vi "Lockin_Metrics.vi"() -> ()   [LabVIEW 2019]
uses:
  src/Instrument.DAQ/Typedefs/DAQ.Sampling.Sampling--Cluster.ctl
  src/Instrument.Lockin/Instrument.Lockin.lvclass
  src/Instrument.Lockin/Typedefs/Results Type--Enum.ctl
  src/Instrument.DAQ/Instrument.DAQ.lvclass
panel:
  in  "Fs":dbl[](array[numeric])=[204800.0, 180000.0, 160000.0, 140000.0, 120000.0, 102400.0, 90000.0, 80000.0, 70000.0, 60000.0, 51200.0, 40000.0, 30000.0, 25600.0, 20000.0, 15000.0, 12800.0]
  out "N":i32=97280
  out "XY Graph 4":cluster{dbl[], dbl[]}[](graph)
  out "XY Graph 3":cluster{dbl[], i32[]}[](graph)
  in  "N start":dbl=102400.0
  in  "N end":dbl=20480.0
  in  "N step":dbl=5120.0
  out "XY Graph 2":cluster{i32[], dbl[]}[](graph)
  in  "stop":bool
  out "Frequency (Hz)":dbl=100.0
  out "XY Graph":cluster{dbl[], dbl[]}[](graph)
  in  "f step":dbl=0.1
  in  "f end":dbl=3.5
  in  "f start":dbl=3.3
  # "Sweep frequency:"
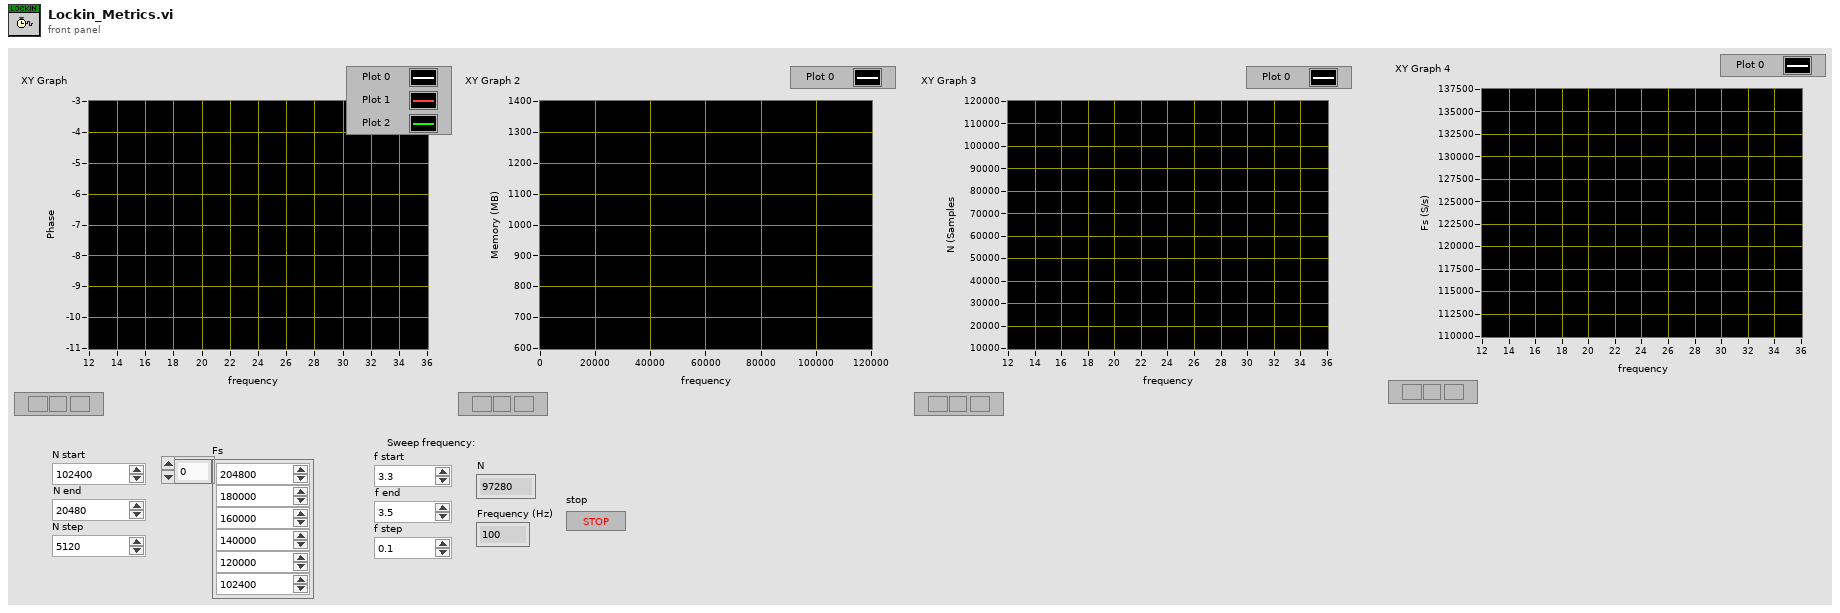
[diagram p1: front panel]
types:
  T1 = typedef "Instrument.Lockin.lvlib/Instrument.DAQ.lvclass/DAQ.Sampling.Sampling--Cluster.ctl" = cluster{"Fs":dbl, "#s":i32}
  T2 = typedef "Instrument.Lockin.lvlib/Instrument.Lockin.lvclass/Results Type--Enum.ctl" = enum16{"X", "Y", "R", "Theta", "Mean"}
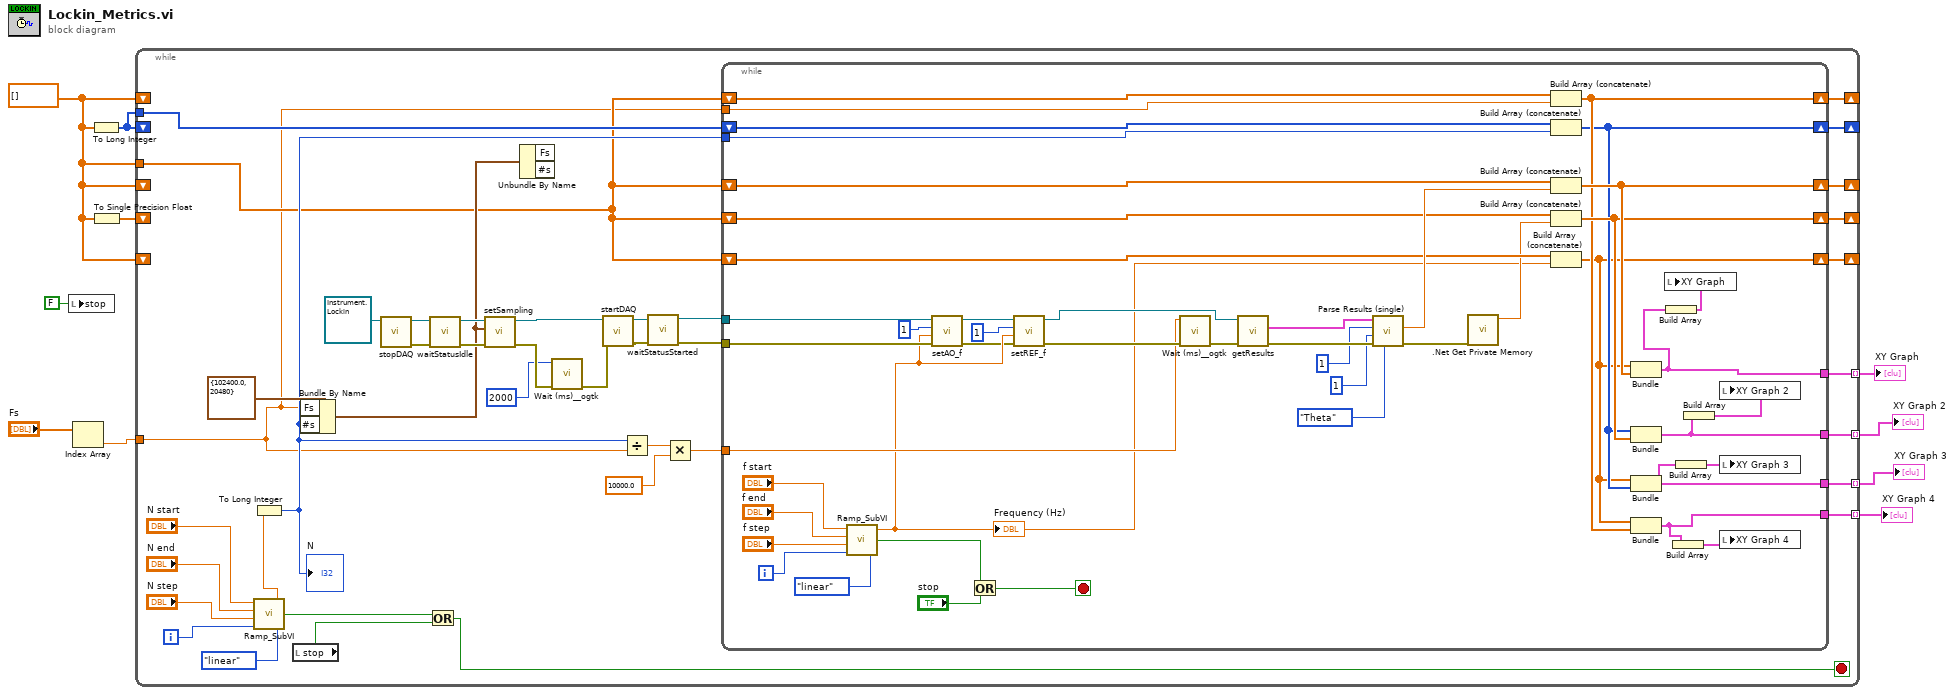
[diagram p0: block diagram]
diagram:
  w7 = dbl[] []
  n1 = local write "stop"(FALSE ("stop")) -> ()
  n2 = Index Array(array="Fs") -> (element=w5:dbl)  [unwired: 1 in]
  n3 = To Long Integer(number=w7) -> (32bit integer=w1:i32[])
  n4 = To Single Precision Float(number=w7) -> (single precision float=w9:sgl[])
  n5 = while {
    shift-right: [w42] -> _
    shift-left: w7 -> [_]
    shift-right: [w39] -> _
    shift-left: w1 -> [_]
    shift-right: [w38] -> _
    shift-left: w7 -> [_]
    shift-right: [w40] -> _
    shift-left: w7 -> [_]
    shift-right: [w41] -> _
    shift-left: w9 -> [_]
    tunnel: [w37] -> w8 mode=indexing
    tunnel: w7 -> [w15]
    tunnel: w5 -> [w14]
    tunnel: [w19] -> w2 mode=indexing
    tunnel: [w18] -> w3 mode=indexing
    tunnel: [w17] -> w4 mode=indexing
    tunnel: w1 -> [w16]
    i -> [w46]
    stop <- w36 stop-if-true
    n6 = call <userlib>:"Ramp_SubVI.vi"("Enum"=enum16{"linear", "power"}."linear", "index"=w46, "step"="N step", "end"="N end", "start"="N start") -> ("Stop?"=w45:bool, "Numeric"=w32:dbl)
    n7 = To Long Integer(number=w32) -> (32bit integer=w31:i32)
    "N" <- w31
    n8 = local read "stop"() -> (w44:bool)
    n9 = Bundle By Name(cluster=T1 {"Fs"=102400.0, "#s"=20480} ("Sampling"), "Fs"=w14, "#s"=w31) -> (w20:T1)
    n10 = call-dynamic "stopDAQ.vi"("Instrument.Lockin in"=refnum<class "Instrument.Lockin.lvclass"> refnum) -> ("error out"=w29:errorcluster, "Instrument.Lockin out"=w30:refnum<class "Instrument.Lockin.lvclass">)  [unwired: 9 in]
    n11 = Or(x=w45, y=w44) -> (x .or. y?=w36:bool)
    n12 = call-dynamic "waitStatusIdle.vi"("error in (no error)"=w29, "Instrument.Lockin in"=w30) -> ("error out"=w28:errorcluster, "Instrument.Lockin out"=w27:refnum<class "Instrument.Lockin.lvclass">)  [unwired: 8 in]
    n13 = call-dynamic "setSampling.vi"("error in (no error)"=w28, "sampling"=w20, "Instrument.Lockin in"=w27) -> ("error out"=w13:errorcluster, "Instrument.Lockin out"=w26:refnum<class "Instrument.Lockin.lvclass">)  [unwired: 7 in]
    n14 = Unbundle By Name(w20) -> ()  [unwired: 2 out]
    n15 = call <userlib>:"Wait (ms)__ogtk.vi"("error in (no error)"=w13, "milliseconds to wait"=u32 2000) -> ("error out"=w12:errorcluster)  [unwired: 8 in, 1 out]
    n16 = call-dynamic "startDAQ.vi"("error in (no error)"=w12, "Instrument.Lockin in"=w26) -> ("error out"=w24:errorcluster, "Instrument.Lockin out"=w25:refnum<class "Instrument.Lockin.lvclass">)  [unwired: 8 in]
    n17 = Divide(x=w31, y=w14) -> (x/y=w35:dbl)
    n18 = call-dynamic "waitStatusStarted.vi"("error in (no error)"=w24, "Instrument.Lockin in"=w25) -> ("error out"=w21:errorcluster, "Instrument.Lockin out"=w22:refnum<class "Instrument.Lockin.lvclass">)  [unwired: 8 in]
    n19 = Multiply(x=w35, y=10000.0) -> (x*y=w33:dbl)
    n20 = while {
      shift-right: [w73] -> w38
      shift-left: w15 -> [w88]
      shift-right: [w85] -> w40
      shift-left: w15 -> [w89]
      shift-right: [w84] -> w41
      shift-left: w15 -> [w86]
      shift-right: [w80] -> w42
      shift-left: w15 -> [w81]
      shift-right: [w77] -> w39
      shift-left: w16 -> [w82]
      tunnel: w21 -> [w78]
      tunnel: w22 -> [w79]
      tunnel: w31 -> [w83]
      tunnel: [w58] -> w37
      tunnel: w33 -> [w71]
      tunnel: [w57] -> w19
      tunnel: [w54] -> w18
      tunnel: [w53] -> w17
      tunnel: w14 -> [w51]
      i -> [w97]
      stop <- w76 stop-if-true
      n21 = call <userlib>:"Ramp_SubVI.vi"("Enum"=enum16{"linear", "power"}."linear", "index"=w97, "step"="f step", "end"="f end", "start"="f start") -> ("Stop?"=w91:bool, "Numeric"=w70:dbl)
      "Frequency (Hz)" <- w70
      n22 = call-dynamic "setAO_f.vi"("error in (no error)"=w78, "Frequency (Hz)"=w70, "AO Channel"=1, "Instrument.Lockin in"=w79) -> ("error out"=w68:errorcluster, "Instrument.Lockin out"=w67:refnum<class "Instrument.Lockin.lvclass">)  [unwired: 6 in]
      n23 = Or(x=w91, y="stop") -> (x .or. y?=w76:bool)
      n24 = call-dynamic "setREF_f.vi"("error in (no error)"=w68, "Frequency (Hz)"=w70, "REF Channel"=1, "Instrument.Lockin in"=w67) -> ("error out"=w74:errorcluster, "Instrument.Lockin out"=w75:refnum<class "Instrument.Lockin.lvclass">)  [unwired: 6 in]
      n25 = call <userlib>:"Wait (ms)__ogtk.vi"("error in (no error)"=w74, "milliseconds to wait"=w71) -> ("error out"=w65:errorcluster)  [unwired: 8 in, 1 out]
      n26 = call-dynamic "getResults.vi"("error in (no error)"=w65, "Instrument.Lockin in"=w75) -> ("error out"=w63:errorcluster, "Results (Dictionary)"=w64:cluster{"key":string, "value":dbl}[])  [unwired: 6 in, 2 out]
      n27 = call "Parse Results (single).vi"("Datatype"=Results_Type--Enum."Theta" ("Type"), "error in (no error)"=w63, "Reference Channel"=1, "AI Channel"=1, "Results (Dictionary)"=w64) -> ("error out"=w59:errorcluster, "Data"=w90:dbl)  [unwired: 3 in, 2 out]
      n28 = call ".Net Get Private Memory.vi"("error in (no error)"=w59) -> ("Private Memory (MB)"=w87:sgl)  [unwired: 9 in, 1 out]
      n29 = Build Array (concatenate)(w81, w51) -> (w80:dbl[])
      n30 = Build Array (concatenate)(w82, w83) -> (w77:i32[])
      n31 = Build Array (concatenate)(w89, w90) -> (w85:dbl[])
      n32 = Build Array (concatenate)(w86, w87) -> (w84:dbl[])
      n33 = Build Array (concatenate)(w88, w70) -> (w73:dbl[])
      n34 = Bundle(w73, w85) -> (w58:cluster{dbl[], dbl[]})  [unwired: 1 in]
      n35 = Bundle(w77, w84) -> (w57:cluster{i32[], dbl[]})  [unwired: 1 in]
      n36 = Bundle(w73, w77) -> (w54:cluster{dbl[], i32[]})  [unwired: 1 in]
      n37 = Bundle(w73, w80) -> (w53:cluster{dbl[], dbl[]})  [unwired: 1 in]
      n38 = Build Array(w58) -> (w72:cluster{dbl[], dbl[]}[])
      n39 = local write "XY Graph"(w72) -> ()
      n40 = Build Array(w53) -> (w52:cluster{dbl[], dbl[]}[])
      n41 = Build Array(w54) -> (w55:cluster{dbl[], i32[]}[])
      n42 = Build Array(w57) -> (w56:cluster{i32[], dbl[]}[])
      n43 = local write "XY Graph 2"(w56) -> ()
      n44 = local write "XY Graph 3"(w55) -> ()
      n45 = local write "XY Graph 4"(w52) -> ()
    }
  }
  "XY Graph" <- w8
  "XY Graph 2" <- w2
  "XY Graph 4" <- w4
  "XY Graph 3" <- w3
